vi "ROS_Topic_Init.vi"(2 "node":string, 3 "topic":string="/robot/head/command_head_nod") -> (1 "ROS out":T1)   [LabVIEW 2010]
doc: "Initializes a topic and returns a ROS cluster. Required before any read or write call."
uses:
  <userlib>/ROSforLV_0.1/ROS/Code/SubVIs/_ROSControl.ctl
  <userlib>/ROSforLV_0.1/ROS/Code/SubVIs/_ROSDirection.ctl
  <userlib>/ROSforLV_0.1/ROS/Code/_ROSDefinition.vi
panel:
  out "Already connected?":bool
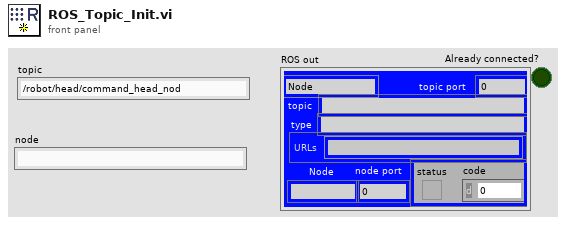
[diagram p1: front panel]
types:
  T1 = typedef "_ROSControl.ctl" = cluster{"topic port":u16, "Node":string, "topic":string, "type":string, "node port":u32, "error ":errorcluster, "Direction":T2, "APIs":string[]}
  T2 = typedef "_ROSDirection.ctl" = enum16{"Node", "Publisher", "Subscriber", "Service Client"}
  T3 = enum32{"Bad", "Idle", "Run top level", "Running"}
  T4 = cluster{"server vi":string, "reference":refnum<vi>, "Description":string[]}[]
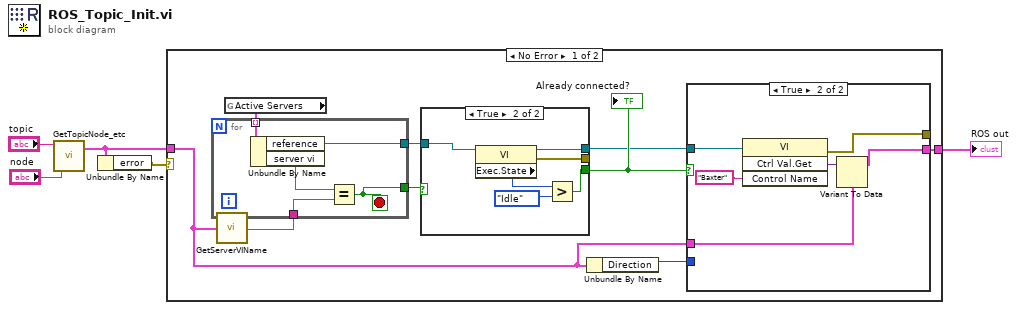
[diagram p0: block diagram]
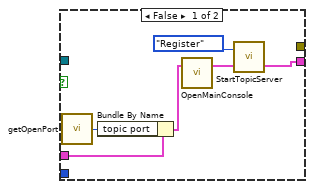
[diagram p2: hidden frame]
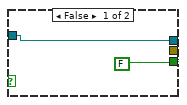
[diagram p3: hidden frame]
diagram:
  n1 = call <userlib>:"GetTopicNode_etc.vi"("node"="node", "topic"="topic") -> ("Baxter"=w1:T1)  [unwired: 1 in]
  n2 = Unbundle By Name(w1) -> ("error"=w2:errorcluster)
  n3 = case shown="No Error" w2 {
    tunnel: [w14 w40] -> w5
    tunnel: w1 -> [w6 w40]
    frame No Error {
      n4 = call <userlib>:"GetServerVIName.vi"("Baxter"=w6) -> ("vi name"=w12:string)
      n5 = global read "_ROSDefinition.vi" "Active Servers"() -> (w13:T4)
      n6 = for {
        tunnel: w13 -> [w39] mode=indexing
        tunnel: w12 -> [w37]
        tunnel: [w36] -> w10
        tunnel: [w35] -> w7
        stop <- w36 stop-if-true
        n7 = Unbundle By Name(w39) -> ("reference"=w35:refnum<vi>, "server vi"=w38:string)
        n8 = Equal?(x=w38, y=w37) -> (x = y?=w36:bool)
      }
      n9 = case shown="True" w10 {
        tunnel: w7 -> [w27 w34]
        tunnel: [FALSE w30] -> w11
        tunnel: [w27 w29] -> w8
        tunnel: [_ w31] -> _
        frame False {
        }
        frame True {
          n10 = property class="VI"(reference=w34) -> (reference out=w29:refnum<vi>, error out=w31:errorcluster, "Exec.State"=w33:T3)  [unwired: 1 in]
          n11 = Greater?(x=w33, y=T3."Idle") -> (0:w30:bool)
        }
      }
      "Already connected?" <- w11
      n12 = Unbundle By Name(w6) -> ("Direction"=w9:T2)
      n13 = case shown="True" w11 {
        tunnel: [w20 w22] -> w14
        tunnel: w9 -> [_ _]
        tunnel: w6 -> [w16 w23]
        tunnel: w8 -> [_ w24]
        tunnel: [_ w21] -> _
        frame False {
          n14 = call <userlib>:"getOpenPort.vi"() -> ("port"=w17:u16)
          n15 = Bundle By Name(cluster=w16, "topic port"=w17) -> (w15:T1)
          n16 = call <userlib>:"OpenMainConsole.vi"("Baxter in"=w15) -> ("Baxter out"=w18:T1)  [unwired: 2 in]
          n17 = call <userlib>:"StartTopicServer.vi"("Baxter in"=w18, "Registration"=enum16{"Register", "Unregister"}."Register") -> ("Baxter out"=w20:T1)  [unwired: 1 in]
        }
        frame True {
          n18 = invoke class="VI" method="Ctrl Val.Get"(reference=w24, "Control Name"="Baxter") -> (error out=w21:errorcluster, "Get Control Value Variant"=w26:variant)  [unwired: 2 in, 2 out]
          n19 = Variant To Data(Variant=w26, type=w23) -> (data=w22:T1)  [unwired: 1 in, 1 out]
        }
      }
    }
    frame Error {
    }
  }
  "ROS out" <- w5
